vi "HardwareLoop.vi"(8 "Error In":errorcluster, 9 "ABLE Configuration":T1, 10 "ABLE Data Structures":T7, 11 "Action Queues":T8) -> (0 "Error Out":errorcluster)   [LabVIEW 2012]
uses:
  ActionQueues.ctl
  UIActionQueueElement.ctl
  UIAction.ctl
  HardwareActionQueueElement.ctl
  HardwareAction.ctl
  ExperimentActionQueueElement.ctl
  ExperimentAction.ctl
  AlarmQueueElement.ctl
  AlarmAction.ctl
  ABLEDataStructures.ctl
  HardwareDisplayData.ctl
  BPM.ctl
  ExperimentHardwareData.ctl
  ExperimentData.ctl
  AlarmData.ctl
  AlarmDatum.ctl
  ABLEConfiguration.ctl
  DisplayConfiguration.ctl
  FolderConfiguration.ctl
  AlarmsConfiguration.ctl
  Keithley6485Configuration.ctl
  Keithley6482Configuration.ctl
  HardwareCollectData.ctl
  PXI6229Data.ctl
  CurrentMeterData.ctl
  PXI6229ActionQueueElement.ctl
  PXI6229Action.ctl
  CurrentMeterQueueElement.ctl
  CurrentMeterAction.ctl
  HardwareLogActionQueueElement.ctl
  HardwareLogAction.ctl
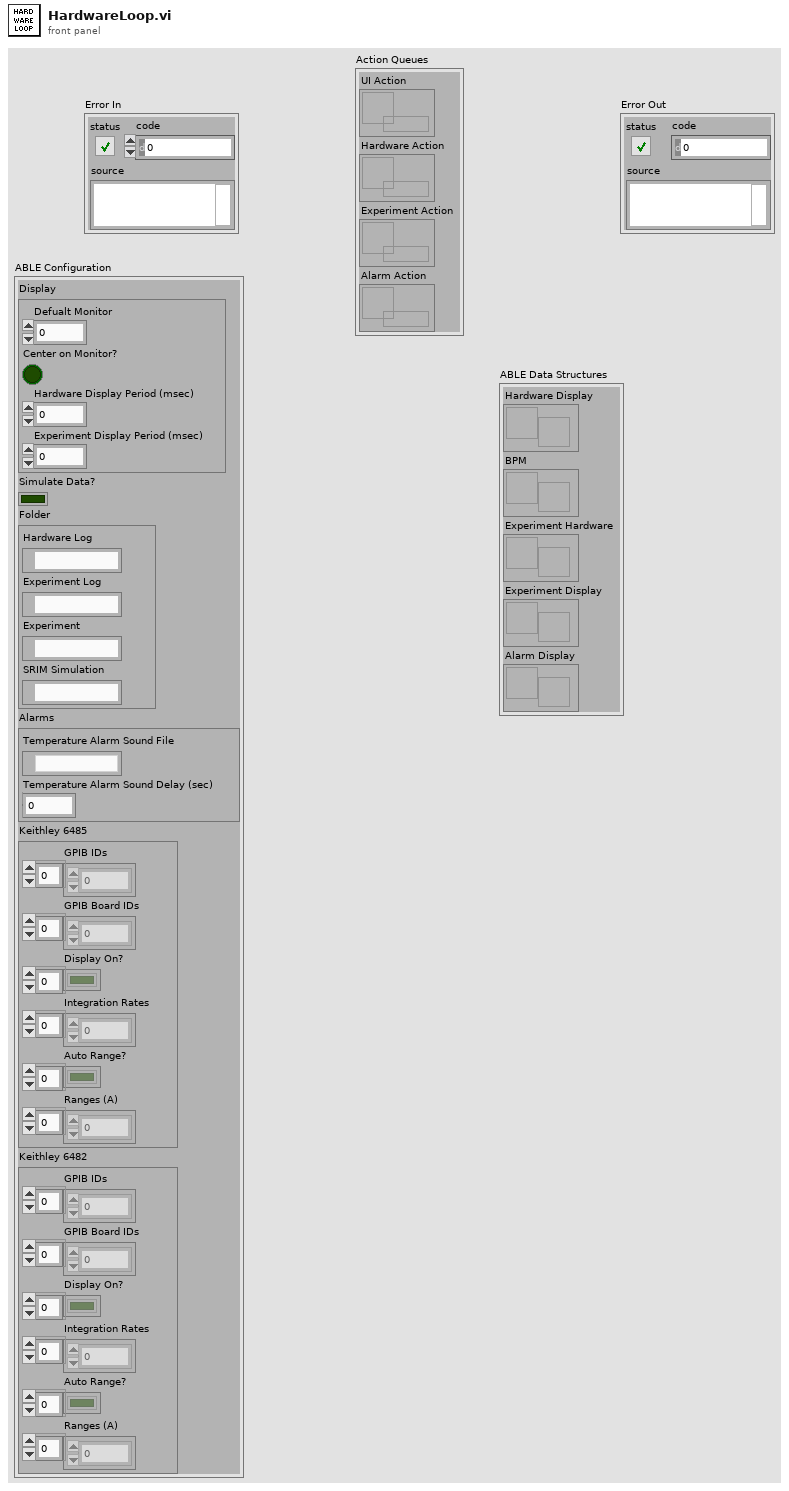
[diagram p1: front panel]
types:
  T1 = typedef "ABLEConfiguration.ctl" = cluster{"Display":T2, "Simulate Data?":bool, "Folder":T3, "Alarms":T4, "Keithley 6485":T5, "Keithley 6482":T6}
  T2 = typedef "DisplayConfiguration.ctl" = cluster{"Defualt Monitor":u16, "Center on Monitor?":bool, "Hardware Display Period (msec)":u32, "Experiment Display Period (msec)":u32}
  T3 = typedef "FolderConfiguration.ctl" = cluster{"Hardware Log":path, "Experiment Log":path, "Experiment":path, "SRIM Simulation":path}
  T4 = typedef "AlarmsConfiguration.ctl" = cluster{"Temperature Alarm Sound File":path, "Temperature Alarm Sound Delay (sec)":dbl}
  T5 = typedef "Keithley6485Configuration.ctl" = cluster{"GPIB IDs":u8[], "GPIB Board IDs":u8[], "Display On?":bool[], "Integration Rates":dbl[], "Auto Range?":bool[], "Ranges (A)":dbl[]}
  T6 = typedef "Keithley6482Configuration.ctl" = cluster{"GPIB IDs":u8[], "GPIB Board IDs":u8[], "Display On?":bool[], "Integration Rates":dbl[], "Auto Range?":bool[], "Ranges (A)":dbl[]}
  T7 = typedef "ABLEDataStructures.ctl" = cluster{"Hardware Display":refnum<notifier>, "BPM":refnum<notifier>, "Experiment Hardware":refnum<notifier>, "Experiment Display":refnum<notifier>, "Alarm Display":refnum<notifier>}
  T8 = typedef "ActionQueues.ctl" = cluster{"UI Action":refnum<queue>, "Hardware Action":refnum<queue>, "Experiment Action":refnum<queue>, "Alarm Action":refnum<queue>}
  T9 = typedef "HardwareLogActionQueueElement.ctl" = cluster{"Action":T10, "Data":variant}
  T10 = typedef "HardwareLogAction.ctl" = enum16{"Initialize", "Clear", "Create", "Log", "Stop", "Shutdown"}
  T11 = typedef "HardwareActionQueueElement.ctl" = cluster{"Action":T12, "Data":variant}
  T12 = typedef "HardwareAction.ctl" = enum16{"Initialize", "Collect", "Shutdown"}
  T13 = typedef "CurrentMeterQueueElement.ctl" = cluster{"Action":T14, "Data":variant}
  T14 = typedef "CurrentMeterAction.ctl" = enum16{"Initialize", "Read", "Simulate", "Error", "Shutdown"}
  T15 = typedef "PXI6229ActionQueueElement.ctl" = cluster{"Action":T16, "Data":variant}
  T16 = typedef "PXI6229Action.ctl" = enum16{"Initialize", "Read", "Simulate", "Error", "Shutdown"}
  T17 = typedef "HardwareCollectData.ctl" = cluster{"PXI-6229 Data":T18, "Current Meter Data":T19}
  T18 = typedef "PXI6229Data.ctl" = cluster{"Temperatures":dbl[][], "Terminal Voltage":dbl[][], "BPM":dbl[][]}
  T19 = typedef "CurrentMeterData.ctl" = dbl[]
  T20 = typedef "HardwareDataStructures.ctl" = cluster{"PXI-6229 Data":refnum<notifier>, "Current Meter Data":refnum<notifier>, "Hardware Log Data":refnum<queue>}
  T21 = typedef "HardwareActionQueues.ctl" = cluster{"PXI-6229 Action":refnum<queue>, "Current Meters Action":refnum<queue>, "Log Action":refnum<queue>}
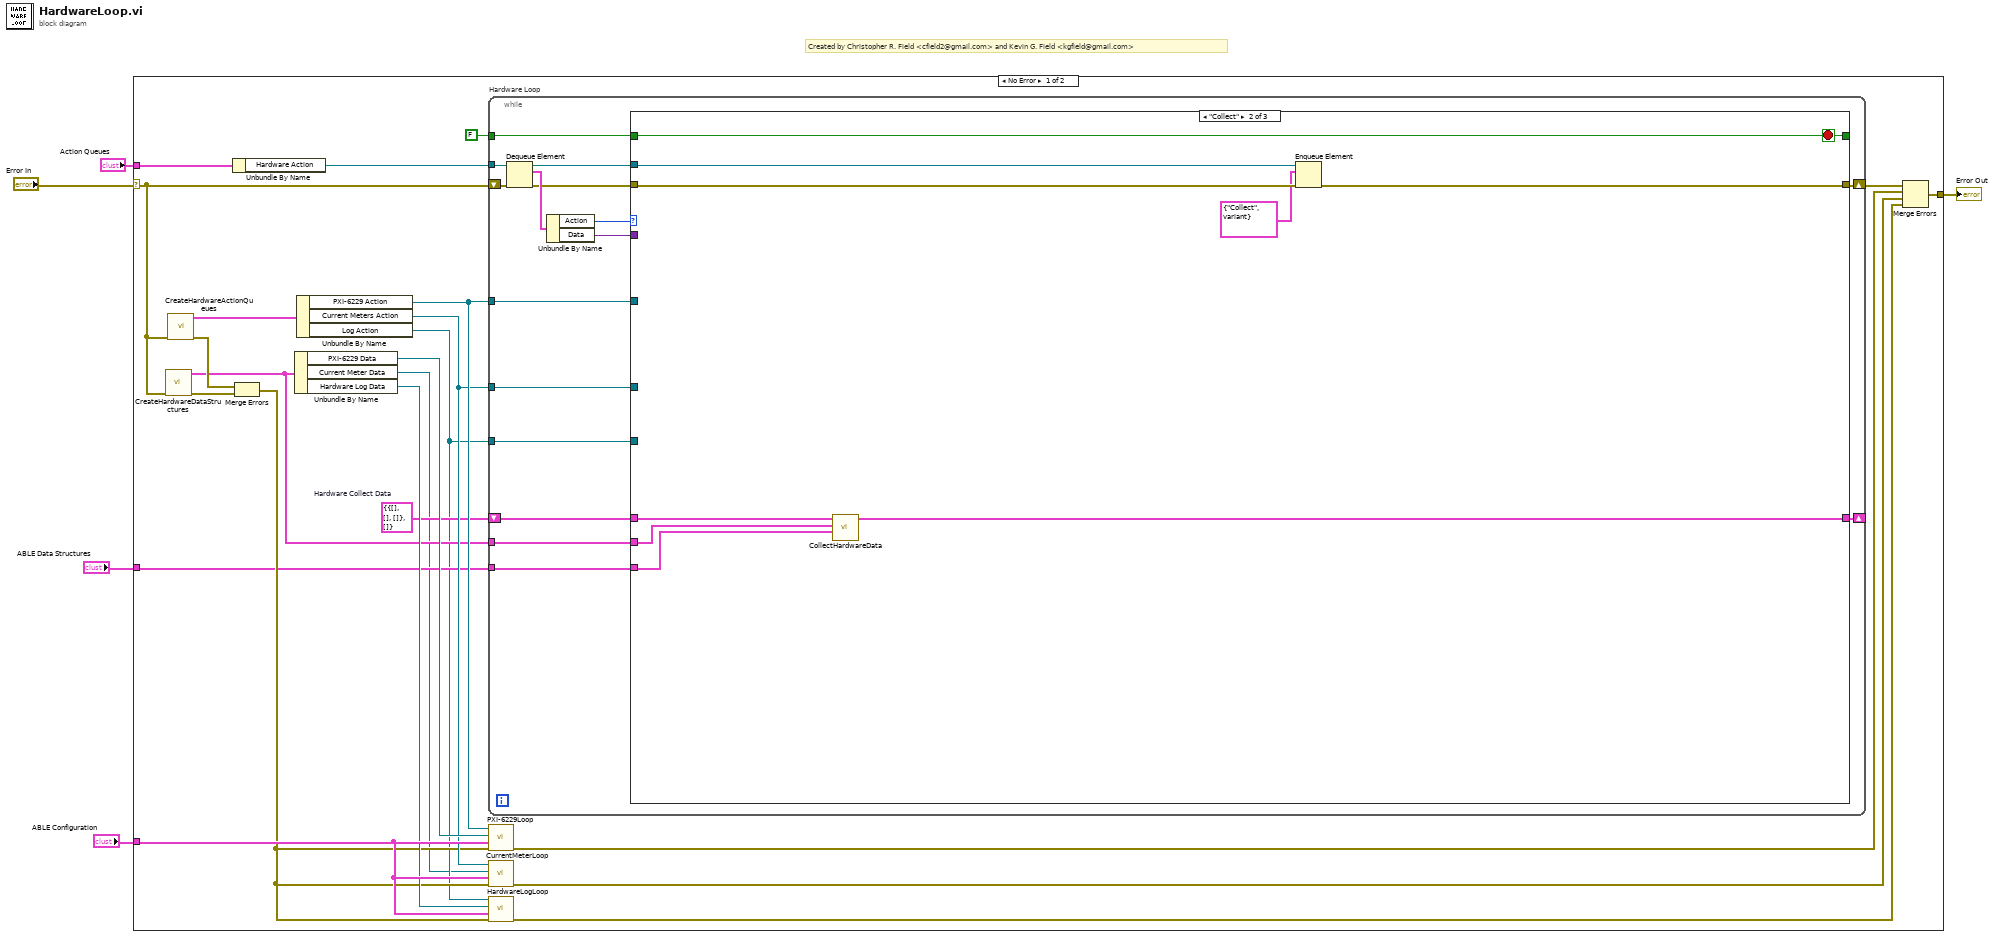
[diagram p0: block diagram]
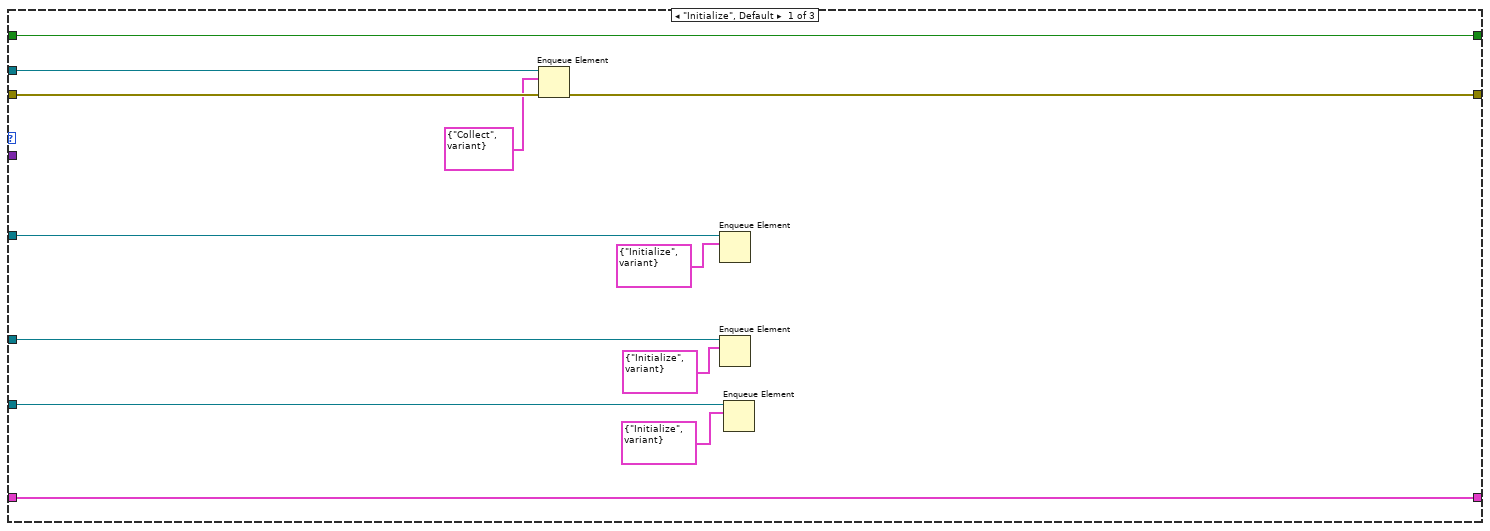
[diagram p2: hidden frame]
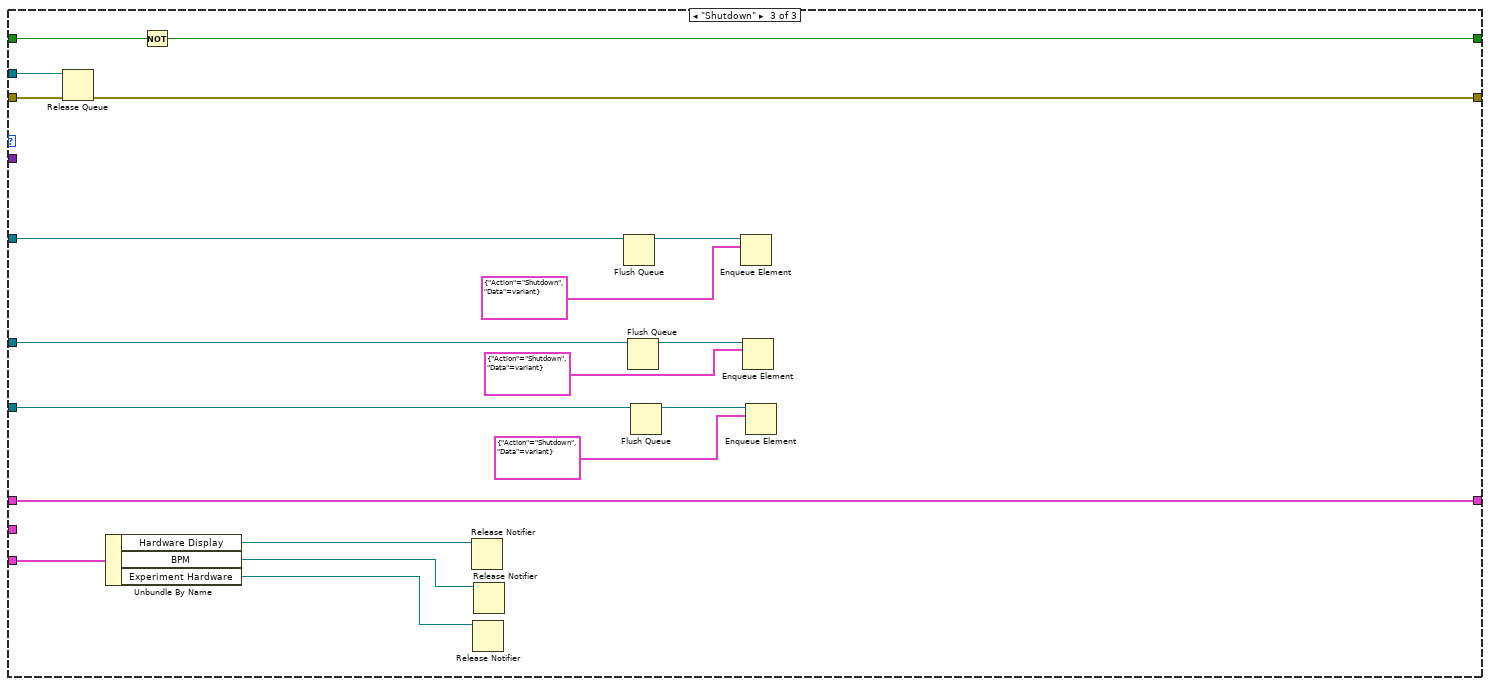
[diagram p3: hidden frame]
diagram:
  # "Created by Christopher R. Field <cfield2@gmail.com> and Kevin G. Field <kgfield@gmail.com>"
  n1 = case shown="No Error" "Error In" {
    selector: "Error In" -> [w21 w86]
    tunnel: [w28 w86] -> w5
    tunnel: "Action Queues" -> [w24 _]
    tunnel: "ABLE Data Structures" -> [w8 _]
    tunnel: "ABLE Configuration" -> [w25 _]
    frame No Error {
      w10 = T17 {"PXI-6229 Data"={"Temperatures"=[], "Terminal Voltage"=[], "BPM"=[]}, "Current Meter Data"=[]}  # Hardware Collect Data
      n2 = call "CreateHardwareDataStructures.vi"("Error In"=w21) -> ("Error Out"=w16:errorcluster, "Hardware Data Structures"=w9:T20)  [unwired: 9 in]
      n3 = call "CreateHardwareActionQueues.vi"("Error In"=w21) -> ("Error Out"=w17:errorcluster, "Hardware Action Queues"=w20:T21)  [unwired: 9 in]
      n4 = Unbundle By Name(w24) -> ("Hardware Action"=w27:refnum<queue>)
      n5 = Merge Errors(w17, w16) -> (w15:errorcluster)
      n6 = Unbundle By Name(w9) -> ("PXI-6229 Data"=w23:refnum<notifier>, "Current Meter Data"=w6:refnum<notifier>, "Hardware Log Data"=w22:refnum<queue>)
      n7 = Unbundle By Name(w20) -> ("PXI-6229 Action"=w19:refnum<queue>, "Current Meters Action"=w18:refnum<queue>, "Log Action"=w7:refnum<queue>)
      n8 = while "Hardware Loop" {
        shift-right: [w39] -> w14
        shift-left: w21 -> [w45]
        tunnel: w19 -> [w37]
        tunnel: w18 -> [w36]
        tunnel: w27 -> [w35]
        tunnel: FALSE -> [w34]
        shift-right: [w31] -> _
        shift-left: w10 -> [w33]
        tunnel: w9 -> [w32]
        tunnel: w8 -> [w30]
        tunnel: w7 -> [w29]
        stop <- w40 stop-if-true
        n9 = Dequeue Element(queue=w35, error in (no error)=w45) -> (queue out=w41:refnum<queue>, element=w44:T11, error out=w42:errorcluster)  [unwired: 1 in, 1 out]
        n10 = Unbundle By Name(w44) -> ("Action"=w43:T12, "Data"=w38:variant)
        n11 = case shown="\"Collect\"" w43 {
          tunnel: w42 -> [w51 w64 w79]
          tunnel: w41 -> [w52 w65 w80]
          tunnel: [w53 w66 w85] -> w40
          tunnel: [w49 w63 w78] -> w39
          tunnel: w38 -> [_ _ _]
          tunnel: w37 -> [w57 _ w76]
          tunnel: w36 -> [w55 _ w75]
          tunnel: w34 -> [w53 w66 w82]
          tunnel: w33 -> [w46 w61 w71]
          tunnel: w32 -> [_ w60 _]
          tunnel: [w46 w59 w71] -> w31
          tunnel: w30 -> [_ w58 w70]
          tunnel: w29 -> [w47 _ w73]
          frame "Initialize", Default {
            n12 = Enqueue Element(queue=w52, element=T11 {"Action"=enum."Collect", "Data"=variant}, error in (no error)=w51) -> (error out=w49:errorcluster)  [unwired: 1 in, 2 out]
            n13 = Enqueue Element(queue=w57, element=T15 {"Action"=enum."Initialize", "Data"=variant}) -> ()  [unwired: 2 in, 3 out]
            n14 = Enqueue Element(queue=w55, element=T13 {"Action"=enum."Initialize", "Data"=variant}) -> ()  [unwired: 2 in, 3 out]
            n15 = Enqueue Element(queue=w47, element=T9 {"Action"=enum."Initialize", "Data"=variant}) -> ()  [unwired: 2 in, 3 out]
          }
          frame "Collect" {
            n16 = call "CollectHardwareData.vi"("ABLE Data Structures"=w58, "Hardware Data Structures"=w60, "Hardware Collect Data In"=w61) -> ("Hardware Collect Data Out"=w59:T17)  [unwired: 7 in, 1 out]
            n17 = Enqueue Element(queue=w65, element=T11 {"Action"=enum."Collect", "Data"=variant}, error in (no error)=w64) -> (error out=w63:errorcluster)  [unwired: 1 in, 2 out]
          }
          frame "Shutdown" {
            n18 = Release Queue(queue=w80, error in (no error)=w79) -> (error out=w78:errorcluster)  [unwired: 1 in, 2 out]
            n19 = Unbundle By Name(w70) -> ("Hardware Display"=w69:refnum<notifier>, "BPM"=w68:refnum<notifier>, "Experiment Hardware"=w67:refnum<notifier>)
            n20 = Not(x=w82) -> (.not. x?=w85:bool)
            n21 = Release Notifier(notifier=w69) -> ()  [unwired: 2 in, 3 out]
            n22 = Release Notifier(notifier=w67) -> ()  [unwired: 2 in, 3 out]
            n23 = Release Notifier(notifier=w68) -> ()  [unwired: 2 in, 3 out]
            n24 = Flush Queue(queue=w76) -> (queue out=w77:refnum<queue>)  [unwired: 1 in, 2 out]
            n25 = Flush Queue(queue=w75) -> (queue out=w74:refnum<queue>)  [unwired: 1 in, 2 out]
            n26 = Flush Queue(queue=w73) -> (queue out=w72:refnum<queue>)  [unwired: 1 in, 2 out]
            n27 = Enqueue Element(queue=w77, element=T15 {"Action"=enum."Shutdown", "Data"=variant}) -> ()  [unwired: 2 in, 3 out]
            n28 = Enqueue Element(queue=w74, element=T13 {"Action"=enum."Shutdown", "Data"=variant}) -> ()  [unwired: 2 in, 3 out]
            n29 = Enqueue Element(queue=w72, element=T9 {"Action"=enum."Shutdown", "Data"=variant}) -> ()  [unwired: 2 in, 3 out]
          }
        }
      }
      n30 = call "PXI-6229Loop.vi"("Error In"=w15, "ABLE Configuration"=w25, "PXI-6229 Data Notifier"=w23, "PXI-6229 Action Queue"=w19) -> ("Error Out"=w13:errorcluster)  [unwired: 7 in]
      n31 = call "CurrentMeterLoop.vi"("Error In"=w15, "ABLE Configuration"=w25, "Current Meter Data"=w6, "Current Meter Action Queue"=w18) -> ("Error Out"=w12:errorcluster)  [unwired: 7 in]
      n32 = call "HardwareLogLoop.vi"("Error In"=w15, "ABLE Configuration"=w25, "Hardware Log Data"=w22, "Hardware Log Action Queue"=w7) -> ("Error Out"=w11:errorcluster)  [unwired: 7 in]
      n33 = Merge Errors(w14, w13, w12, w11) -> (w28:errorcluster)
    }
    frame Error {
    }
  }
  "Error Out" <- w5
